vi "Send Menu Response.vi"(7 "Message Priority (Normal)":T1=enum."Normal", 8 "error in (no error)":errorcluster, 10 "Menu Tag":string, 11 "Message Enqueuer":refnum<class "Message Enqueuer.lvclass">) -> (0 "error out":errorcluster, 3 "Message Enqueuer out":refnum<class "Message Enqueuer.lvclass">)   [LabVIEW 2023, in "Main.lvlib" / "Menu Response Msg.lvclass"]
doc: "This VI sends the message to an actor."
uses:
  Menu Response Msg.lvclass
  builds/Framework/Actor Framework.lvlibp/1abvi3w/vi.lib/ActorFramework/Message Enqueuer/Message Enqueuer.lvclass
  builds/Framework/Actor Framework.lvlibp/1abvi3w/vi.lib/ActorFramework/Message Enqueuer/Message Priority.ctl
  Menu Response Msg.lvclass/Menu Response Msg.ctl
  C:/Users/Public/Documents/Development/builds/Framework/Actor Framework.lvlibp/1abvi3w/vi.lib/ActorFramework/Message/Message.lvclass
  C:/Users/Public/Documents/Development/Application/Main/Main Messages/Menu Response Msg/Menu Response Msg.lvclass
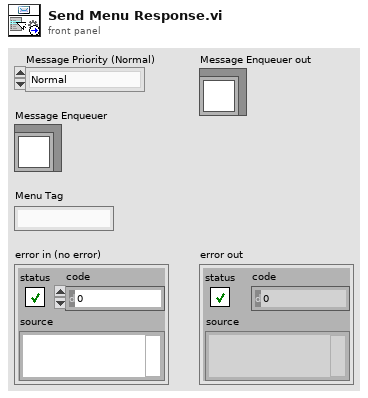
[diagram p1: front panel]
types:
  T1 = typedef "Actor Framework.lvlibp/Message Enqueuer.lvclass/Message Priority.ctl" = enum16{"Low", "Normal", "High"}
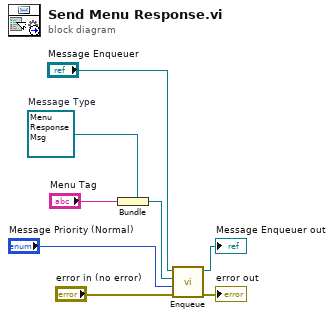
[diagram p0: block diagram]
diagram:
  w5 = refnum<class "Menu Response Msg.lvclass"> refnum  # Message Type
  n1 = Bundle(cluster=w5, "Menu Tag") -> (w4:refnum<class "Menu Response Msg.lvclass">)
  n2 = call "Enqueue.vi"("error in (no error)"="error in (no error)", "Message Priority (Normal)"="Message Priority (Normal)", "Message"=w4, "Message Enqueuer in"="Message Enqueuer") -> ("error out"=→"error out":errorcluster, "Message Enqueuer in"=→"Message Enqueuer out":refnum<class "Message Enqueuer.lvclass">)  [unwired: 6 in]
